vi "Fast Decaying Nanowries.vi"() -> ()   [LabVIEW 2020]
uses:
  <userlib>/LevyLab/XY Utilities/subVIs/Linear Fit (single).vi
  <userlib>/LevyLab/LV to ITX/Data/Data.lvclass
  <userlib>/LevyLab/XY Utilities/xy_utilities.lvlib
panel:
  out "E_a":dbl
  out "ln(300 K Slope)":dbl
  out "ln(275 K slope)":dbl
  out "G4T vs t":T1(graph)
  in  "300 K":path=path "G:/My Drive/ansom/Data/MFP3D/Users/Aaron/SA40144E.20210824/monitor/monitor conductance.000000.dat"
  in  "275 K":path=path "G:/My Drive/ansom/Data/PPMS 2/SA40144.20210824/45-LockinFieldSweep_hash_16_27_stripe/SA40144.20210824.000000.dat"
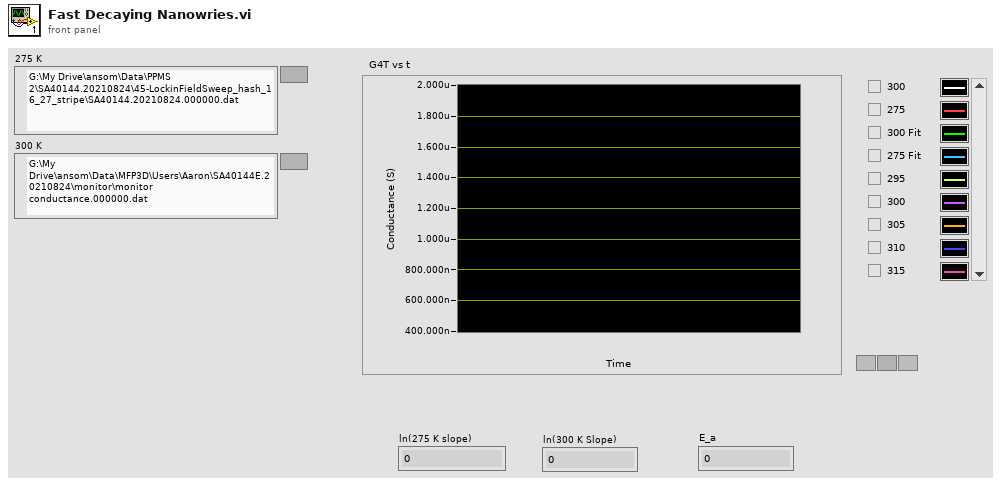
[diagram p1: front panel]
types:
  T1 = cluster{"Data":dbl[], "Best Exponential Fit":dbl[]}[]
  T2 = typedef "Data.lvclass/Dictionary--cluster.ctl" = cluster{"key":string, "value":variant}
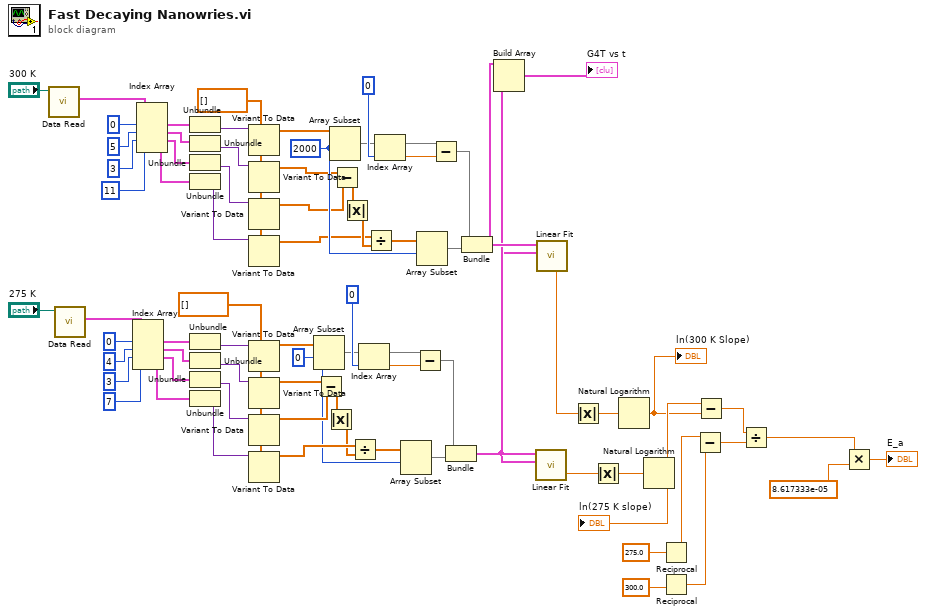
[diagram p0: block diagram]
diagram:
  w24 = 2000 ("index")
  w33 = 0 ("index")
  w52 = dbl[] []
  w51 = dbl[] []
  n1 = call <userlib>:"Data Read.vi"("path"="300 K") -> ("Data (Dictionary)"=w74:T2[])  [unwired: 7 in, 3 out]
  n2 = call <userlib>:"Data Read.vi"("path"="275 K") -> ("Data (Dictionary)"=w73:T2[])  [unwired: 7 in, 3 out]
  n3 = Index Array(array=w73, index #1=0 ("index"), index #2=4 ("index"), index #3=3 ("index"), index #4=7 ("index")) -> (element #1=w60:T2, element #2=w59:T2, element #3=w58:T2, element #4=w57:T2)
  n4 = Index Array(array=w74, index #1=0 ("index"), index #2=5 ("index"), index #3=3 ("index"), index #4=11 ("index")) -> (element #1=w64:T2, element #2=w63:T2, element #3=w62:T2, element #4=w61:T2)
  n5 = Unbundle(w64) -> ("value"=w55:variant)  [unwired: 1 out]
  n6 = Unbundle(w63) -> ("value"=w54:variant)  [unwired: 1 out]
  n7 = Unbundle(w62) -> ("value"=w53:variant)  [unwired: 1 out]
  n8 = Unbundle(w61) -> ("value"=w56:variant)  [unwired: 1 out]
  n9 = Unbundle(w60) -> ("value"=w50:variant)  [unwired: 1 out]
  n10 = Unbundle(w59) -> ("value"=w47:variant)  [unwired: 1 out]
  n11 = Unbundle(w58) -> ("value"=w48:variant)  [unwired: 1 out]
  n12 = Unbundle(w57) -> ("value"=w49:variant)  [unwired: 1 out]
  n13 = Variant To Data(type=w52, Variant=w55) -> (data=w20:dbl[])  [unwired: 1 in, 1 out]
  n14 = Variant To Data(type=w52, Variant=w54) -> (data=w21:dbl[])  [unwired: 1 in, 1 out]
  n15 = Variant To Data(type=w52, Variant=w53) -> (data=w22:dbl[])  [unwired: 1 in, 1 out]
  n16 = Variant To Data(type=w52, Variant=w56) -> (data=w23:dbl[])  [unwired: 1 in, 1 out]
  n17 = Variant To Data(type=w51, Variant=w50) -> (data=w40:dbl[])  [unwired: 1 in, 1 out]
  n18 = Variant To Data(type=w51, Variant=w47) -> (data=w46:dbl[])  [unwired: 1 in, 1 out]
  n19 = Variant To Data(type=w51, Variant=w48) -> (data=w45:dbl[])  [unwired: 1 in, 1 out]
  n20 = Variant To Data(type=w51, Variant=w49) -> (data=w43:dbl[])  [unwired: 1 in, 1 out]
  n21 = Array Subset(array=w40, index=w33) -> (w37:dbl[])  [unwired: 1 in]
  n22 = Subtract(x=w46, y=w45) -> (x-y=w44:dbl[])
  n23 = Absolute Value(x=w44) -> (abs(x)=w41:dbl[])
  n24 = Array Subset(array=w20, index=w24) -> (w28:dbl[])  [unwired: 1 in]
  n25 = Subtract(x=w21, y=w22) -> (x-y=w32:dbl[])
  n26 = Absolute Value(x=w32) -> (abs(x)=w31:dbl[])
  n27 = Divide(x=w43, y=w41) -> (x/y=w35:dbl[])
  n28 = Index Array(array=w37, index=0) -> (element=w39:dbl)
  n29 = Divide(x=w23, y=w31) -> (x/y=w26:dbl[])
  n30 = Index Array(array=w28, index=0) -> (element=w30:dbl)
  n31 = Array Subset(array=w35, index=w33) -> (w34:dbl[])  [unwired: 1 in]
  n32 = Subtract(x=w37, y=w39) -> (x-y=w36:dbl[])
  n33 = Array Subset(array=w26, index=w24) -> (w25:dbl[])  [unwired: 1 in]
  n34 = Subtract(x=w28, y=w30) -> (x-y=w27:dbl[])
  n35 = Bundle(w36, w34) -> (w18:cluster{dbl[], dbl[]})  [unwired: 1 in]
  n36 = Bundle(w27, w25) -> (w19:cluster{dbl[], dbl[]})  [unwired: 1 in]
  n37 = call-poly <userlib>:"Linear Fit.vi"("XY-data"=w18) -> ("Best Fit"=w1:cluster{"X-array":dbl[], "Y-array":dbl[]}, "slope"=w6:dbl)  [unwired: 4 in, 5 out]
  n38 = call-poly <userlib>:"Linear Fit.vi"("XY-data"=w19) -> ("Best Fit"=w2:cluster{"X-array":dbl[], "Y-array":dbl[]}, "slope"=w4:dbl)  [unwired: 4 in, 5 out]
  n39 = Build Array(w19, w18, w2, w1) -> (→"G4T vs t":cluster{"X-array":dbl[], "Y-array":dbl[]}[])
  n40 = Absolute Value(x=w4) -> (abs(x)=w7:dbl)
  n41 = Absolute Value(x=w6) -> (abs(x)=w8:dbl)
  n42 = Natural Logarithm(1:w7) -> (0:w3:dbl)
  "ln(300 K Slope)" <- w3
  n43 = Natural Logarithm(1:w8) -> (0:w5:dbl)
  "ln(275 K slope)" <- w5
  n44 = Reciprocal(x=275.0) -> (1/x=w13:dbl)
  n45 = Reciprocal(x=300.0) -> (1/x=w12:dbl)
  n46 = Subtract(x=w13, y=w12) -> (x-y=w11:dbl)
  n47 = Subtract(x=w5, y=w3) -> (x-y=w10:dbl)
  n48 = Divide(x=w10, y=w11) -> (x/y=w9:dbl)
  n49 = Multiply(x=w9, y=8.617333e-05) -> (x*y=→"E_a":dbl)
